vi "2D_PyArray_to_BW_IMAQ.vi"(6 "Image Name":string="B_", 8 "error in (no error)":errorcluster, 10 "pythonArr_IN":u8[][](array[numeric]), 11 "Refnum in":T1) -> (0 "error out":errorcluster, 2 "output size":i32[](array[numeric]), 3 "Refnum out":T1)   [LabVIEW 2021, in "Framework_lib.lvlib"]
uses:
  SubVis/QMH/Framework_lib.lvlib
  <vilib>/vision/Image Controls.llb/IMAQ Image.ctl
  <vilib>/vision/NI_Vision_Development_Module.lvlib
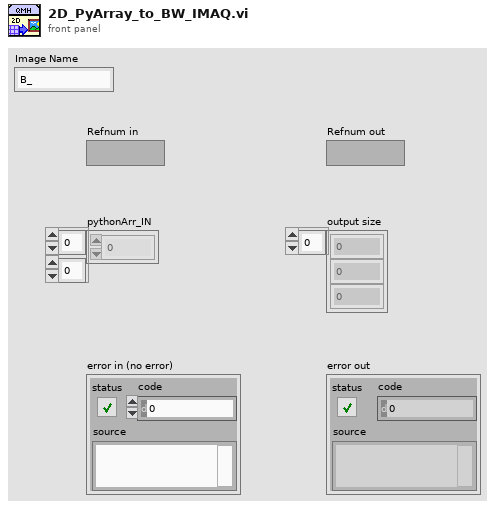
[diagram p1: front panel]
types:
  T1 = typedef "IMAQ Image.ctl" = refnum<image>
  T2 = typedef "Image Type" = u32
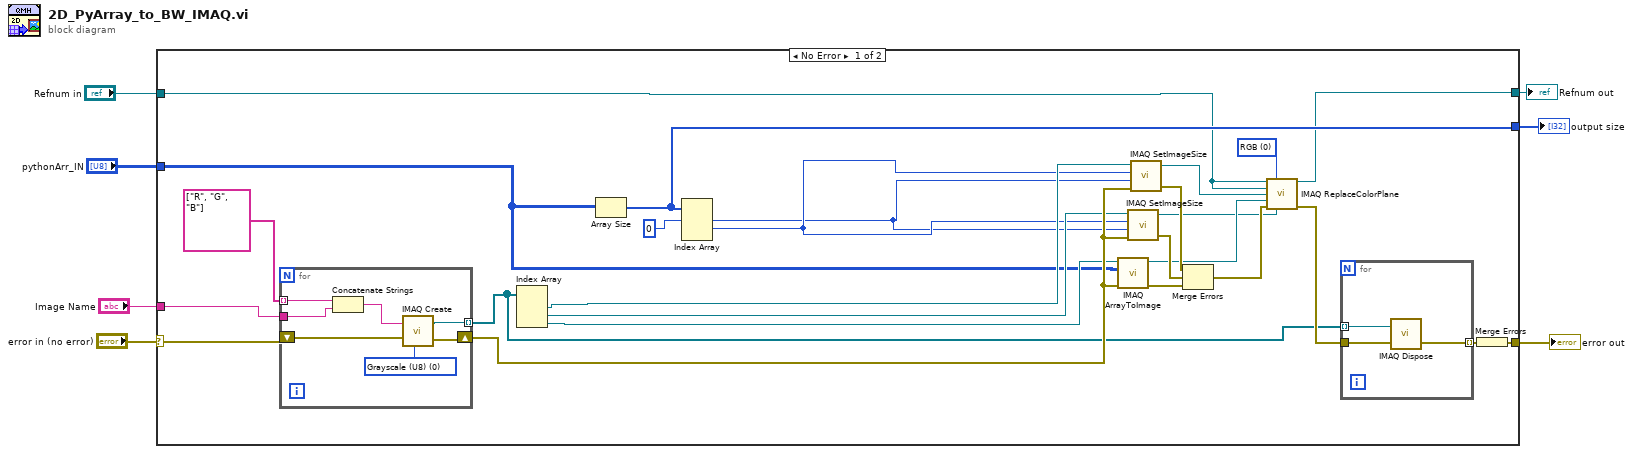
[diagram p0: block diagram]
diagram:
  n1 = case shown="No Error" "error in (no error)" {
    selector: "error in (no error)" -> [w24 w45]
    tunnel: [w26 _] -> w7
    tunnel: [w25 w44] -> w6
    tunnel: [w15 w45] -> w5
    tunnel: "Refnum in" -> [w8 w44]
    tunnel: "pythonArr_IN" -> [w13 _]
    tunnel: "Image Name" -> [w18 _]
    frame No Error {
      w29 = u16 0 items=["RGB", "HSL", "HSV", "HSI"] ("Color Mode")
      n2 = for {
        shift-right: [w41] -> w23
        shift-left: w24 -> [w42]
        tunnel: [w40] -> w14 mode=indexing
        tunnel: string[] ["R", "G", "B"] ("Image Name 2") -> [w39] mode=indexing
        tunnel: w18 -> [w37]
        w43 = T2 0 items=["Grayscale (U8)", "Grayscale (I16)", "Grayscale (SGL)", "Complex (CSG)", "RGB (U32)", "HSL (U32)", "RGB (U64)", "Grayscale (U16)"] ("Image Type")
        n3 = Concatenate Strings(w39, w37) -> (w38:string)
        n4 = call "IMAQ Create"("Image Name"=w38, "Image Type"=w43, "error in (no error)"=w42) -> ("New Image"=w40:T1, "error out"=w41:errorcluster)  [unwired: 2 in]
      }
      n5 = Index Array(array=w14) -> (element #1=w22:T1, element #2=w21:T1, element #3=w20:T1)  [unwired: 3 in]
      n6 = Array Size(array=w13) -> (size(s)=w26:i32[])
      n7 = Index Array(array=w26, index #1=0 ("index")) -> (element #1=w11:i32, element #2=w12:i32)  [unwired: 2 in, 1 out]
      n8 = call "IMAQ ArrayToImage"("error in (no error)"=w23, "Image Pixels (U8)"=w13, "Image"=w20) -> ("error out"=w30:errorcluster, "Image Out"=w10:T1)  [unwired: 7 in]
      n9 = call "IMAQ SetImageSize"("error in (no error)"=w23, "Y Resolution"=w11, "X Resolution"=w12, "Image"=w21) -> ("error out"=w32:errorcluster, "Image Out"=w9:T1)  [unwired: 1 in]
      n10 = call "IMAQ SetImageSize"("error in (no error)"=w23, "Y Resolution"=w11, "X Resolution"=w12, "Image"=w22) -> ("error out"=w33:errorcluster, "Image Out"=w28:T1)  [unwired: 1 in]
      n11 = Merge Errors(w33, w32, w30) -> (w31:errorcluster)
      n12 = call "IMAQ ReplaceColorPlane"("Image Src"=w8, "Color Mode"=w29, "Image Dst"=w8, "Red or Hue Plane"=w28, "Green or Sat Plane"=w10, "error in (no error)"=w31, "Blue or Luma or Val or Inten Plane"=w9) -> ("Image Dst Out"=w25:T1, "error out"=w16:errorcluster)  [unwired: 7 in]
      n13 = for {
        tunnel: [w35] -> w17 mode=indexing
        tunnel: w16 -> [w36]
        tunnel: w14 -> [w34] mode=indexing
        n14 = call "IMAQ Dispose"("Image"=w34, "error in (no error)"=w36) -> ("error out"=w35:errorcluster)  [unwired: 4 in]
      }
      n15 = Merge Errors(w17) -> (w15:errorcluster)
    }
    frame Error {
    }
  }
  "output size" <- w7
  "Refnum out" <- w6
  "error out" <- w5
